vi "GetM.vi"(0 "q":dbl[](array[numeric]), 5 "m":dbl, 7 "L":dbl, 9 "L1":dbl, 11 "I":dbl) -> (8 "M":T1)   [LabVIEW 2019]
uses:
  <vilib>/Analysis/Matrix/Datatypes/RealMatrix.ctl
  <vilib>/Analysis/Matrix/NI_Matrix.lvlib
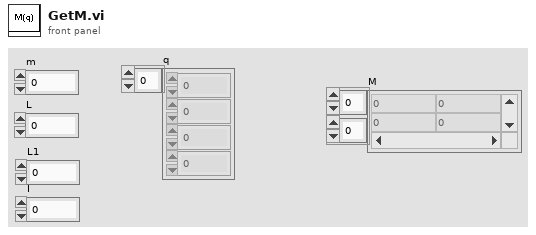
[diagram p1: front panel]
types:
  T1 = typedef "NI_Matrix.lvlib/RealMatrix.ctl" = dbl[][]
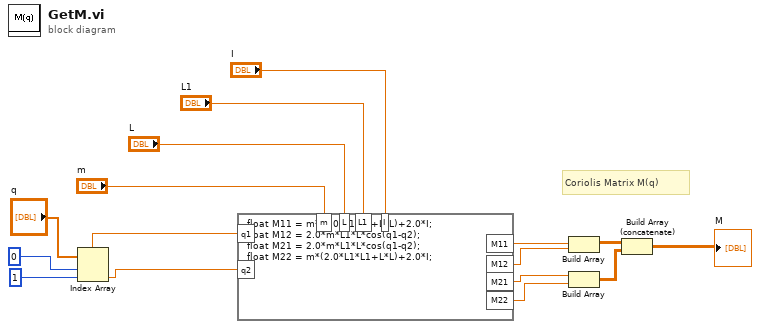
[diagram p0: block diagram]
diagram:
  # "Coriolis Matrix M(q)"
  n1 = Index Array(array="q", index #1=0 ("index (row)"), index #2=1 ("index (col)")) -> (element #1=w14:dbl, element #2=w1:dbl)
  n2 = formula code="float M11 = m*(2.0*L1*L1+L*L)+2.0*I;\nfloat M12 = 2.0*m*L1*L*cos(q1-q2);\nfloat M21 = 2.0*m*L1*L*cos(q1-q2);\nfloat M22 = m*(2.0*L1*L1+L*L)+2.0*I;"("m"="m", "L"="L", "L1"="L1", "q1"=w14, "q2"=w1, "I"="I") -> ("M11"=w6:dbl, "M12"=w5:dbl, "M21"=w4:dbl, "M22"=w3:dbl)
  n3 = Build Array(w6, w5) -> (w9:T1)
  n4 = Build Array(w4, w3) -> (w8:T1)
  n5 = Build Array (concatenate)(w9, w8) -> (→"M":T1)
